vi "daqio_Re-Connect_Device.vi"(6 "re-connect timeouts":u32=1000, 7 "Credentials":T4, 8 "error in":errorcluster, 9 "override any errors":bool, 10 "re-connect attempts":i32=5, 11 "daq.io type in":T2={"daq.io ref"=refnum, "daq.io API Base"="http://dashboard.daq.io/api/v1", "Device Type Key"="", "Device Key"="", "Account ID"="", "online"=FALSE}) -> (0 "error out":errorcluster, 2 "status":T1, 3 "daq.io type out":T2={"daq.io ref"=refnum, "daq.io API Base"="http://dashboard.daq.io/api/v1", "Device Type Key"="", "Device Key"="", "Account ID"="", "online"=FALSE})   [LabVIEW 2013, in "daqio minimal.lvlib"]
doc: "This VI tries to re-connect the current device (the one the VI is executed on) to the daq.io cloud connection.\n\nThis VI can use multiple attempts to re-connect to the cloud. On Vxworks targets such as CompactRIO and SingleBoard RIO systems, this check may result in a timed out http GET function that can block the execution of code, therefore please run it in parallel and share the connection data globally by queue or FGV."
uses:
  daqio minimal.lvlib
  _typedefs/daqio-Credentials.ctl
  _typedefs/daqio-Type.ctl
  <vilib>/httpClient/ClientHandle.ctl
  _typedefs/daqio-reconnect-status.ctl
  <vilib>/httpClient/LabVIEWHTTPClient.lvlib
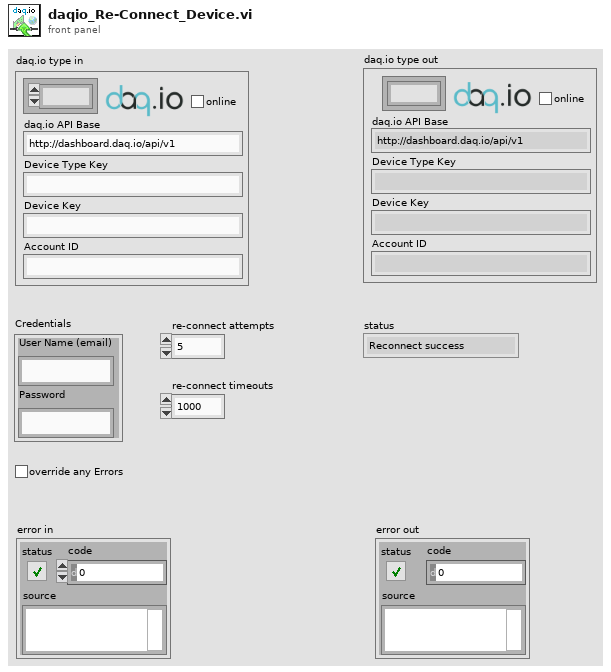
[diagram p1: front panel]
types:
  T1 = typedef "daqio minimal.lvlib/daqio-reconnect-status.ctl" = enum16{"Reconnect success", "Reconnect failed", "Connected"}
  T2 = typedef "daqio minimal.lvlib/daqio-Type.ctl" = cluster{"daq.io ref":T3, "daq.io API Base":string, "Device Type Key":string, "Device Key":string, "Account ID":string, "online":bool}
  T3 = typedef "LabVIEWHTTPClient.lvlib/ClientHandle.ctl" = refnum<k1>
  T4 = typedef "daqio minimal.lvlib/daqio-Credentials.ctl" = cluster{"User Name (email)":string, "Password":string}
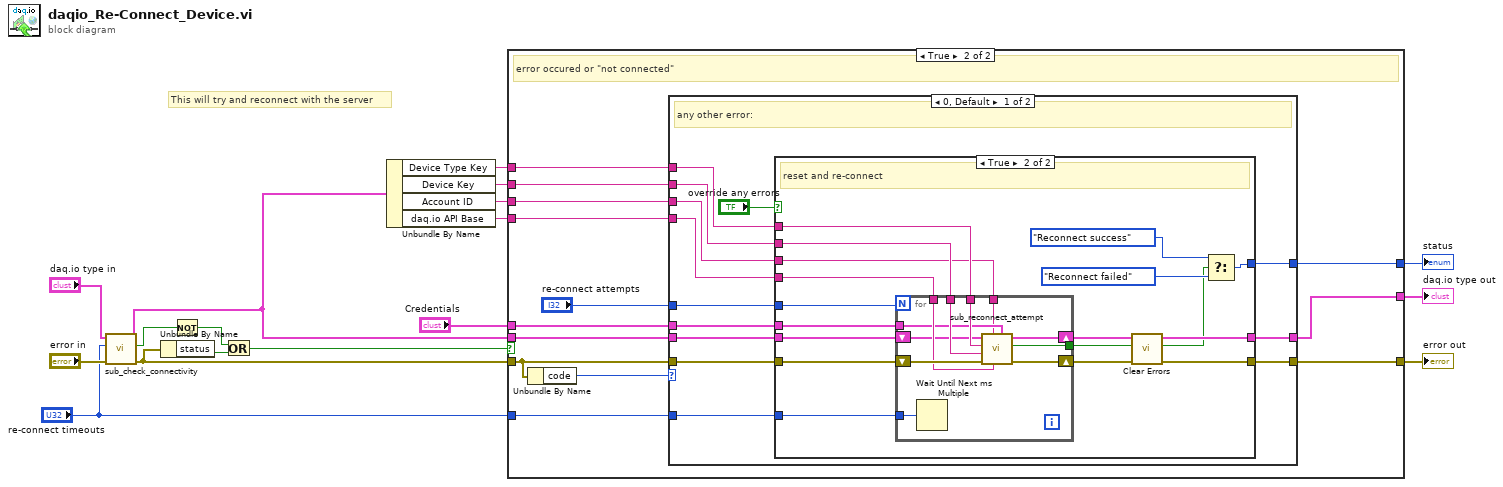
[diagram p0: block diagram]
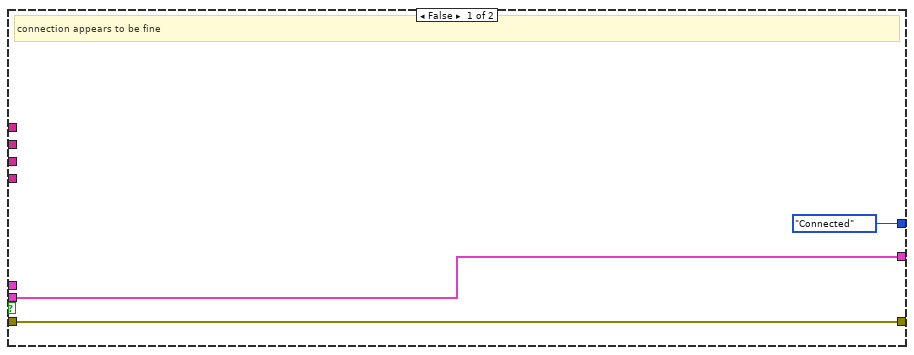
[diagram p2: hidden frame]
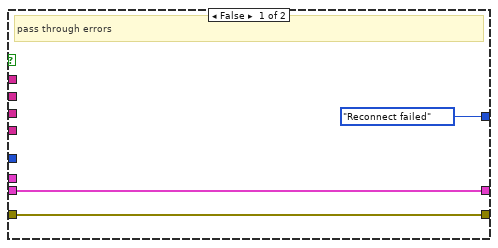
[diagram p3: hidden frame]
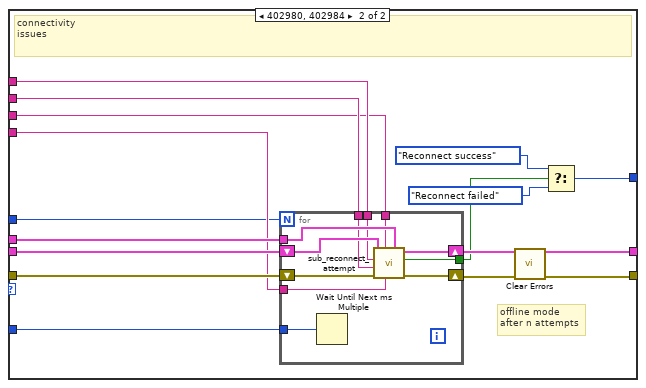
[diagram p4: hidden frame]
diagram:
  # "This will try and reconnect with the server"
  n1 = call "sub_check_connectivity.vi"("error in (no error)"="error in", "timeout (1000)"="re-connect timeouts", "daq.io type in"="daq.io type in") -> ("error out"=w3:errorcluster, "connected"=w2:bool, "daq.io type out"=w5:T2)  [unwired: 6 in]
  n2 = Unbundle By Name(w3) -> ("status"=w14:bool)
  n3 = Not(x=w2) -> (.not. x?=w15:bool)
  n4 = Or(x=w15, y=w14) -> (x .or. y?=w13:bool)
  n5 = Unbundle By Name(w5) -> ("Device Type Key"=w11:string, "Device Key"=w10:string, "Account ID"=w6:string, "daq.io API Base"=w7:string)
  n6 = case shown="True" w13 {
    tunnel: w3 -> [w19 w32]
    tunnel: "Credentials" -> [_ w31]
    tunnel: w11 -> [_ w30]
    tunnel: w10 -> [_ w29]
    tunnel: [w20 w28] -> w9
    tunnel: [w19 w27] -> w8
    tunnel: w5 -> [w20 w26]
    tunnel: w7 -> [_ w25]
    tunnel: w6 -> [_ w24]
    tunnel: [daqio-reconnect-status."Connected" ("status 2") w22] -> w4
    tunnel: "re-connect timeouts" -> [_ w21]
    frame False {
      # "connection appears to be fine"
    }
    frame True {
      # "error occured or \"not connected\""
      n7 = Unbundle By Name(w32) -> ("code"=w33:i32)
      n8 = case shown="0, Default" w33 {
        tunnel: w32 -> [w45 w88]
        tunnel: w31 -> [w44 w91]
        tunnel: w30 -> [w42 w90]
        tunnel: w29 -> [w43 w89]
        tunnel: [w41 w85] -> w28
        tunnel: [w40 w81] -> w27
        tunnel: w26 -> [w39 w92]
        tunnel: w25 -> [w38 w86]
        tunnel: w24 -> [w37 w87]
        tunnel: "re-connect attempts" -> [w36 w84]
        tunnel: w21 -> [w35 w83]
        tunnel: [w34 w82] -> w22
        frame 0, Default {
          # "any other error:"
          n9 = case shown="True" "override any errors" {
            tunnel: w45 -> [w49 w65]
            tunnel: w44 -> [_ w60]
            tunnel: w43 -> [_ w63]
            tunnel: w42 -> [_ w62]
            tunnel: [w48 w58] -> w41
            tunnel: [w49 w54] -> w40
            tunnel: w39 -> [w48 w61]
            tunnel: w38 -> [_ w64]
            tunnel: w37 -> [_ w59]
            tunnel: w36 -> [_ w57]
            tunnel: w35 -> [_ w56]
            tunnel: [daqio-reconnect-status."Reconnect failed" ("status 2") w55] -> w34
            frame False {
              # "pass through errors"
            }
            frame True {
              # "reset and re-connect"
              n10 = for {
                N: w57 -> [_]
                tunnel: w64 -> [w74]
                tunnel: w63 -> [w73]
                tunnel: w62 -> [w72]
                tunnel: w60 -> [w70]
                tunnel: w59 -> [w69]
                tunnel: [w68] -> w50
                shift-right: [w76] -> w51
                shift-left: w65 -> [w75]
                shift-right: [w67] -> w58
                shift-left: w61 -> [w71]
                tunnel: w56 -> [w66]
                n11 = Wait Until Next ms Multiple(millisecond multiple=w66) -> ()  [unwired: 1 out]
                n12 = call "sub_reconnect_attempt.vi"("Credentials"=w70, "daq.io API Base"=w74, "Account ID"=w69, "error in (no error)"=w75, "Device Key"=w73, "Device Type Key"=w72, "daq.io type in OLD"=w71) -> ("error out"=w76:errorcluster, "logged in?"=w68:bool, "daq.io type out"=w67:T2)  [unwired: 2 in]
              }
              n13 = call <vilib>:"Clear Errors.vi"("error in (no error)"=w51) -> ("error out"=w54:errorcluster)  [unwired: 6 in]
              n14 = Select(t=daqio-reconnect-status."Reconnect success" ("status 2"), s=w50, f=daqio-reconnect-status."Reconnect failed" ("status 2")) -> (s? t:f=w55:T1)
            }
          }
        }
        frame 402980, 402984 {
          # "offline mode\nafter n attempts"
          # "connectivity\nissues"
          n15 = for {
            N: w84 -> [_]
            tunnel: w91 -> [w102]
            tunnel: w90 -> [w101]
            tunnel: w89 -> [w100]
            tunnel: w87 -> [w98]
            tunnel: w86 -> [w97]
            tunnel: [w94] -> w77
            shift-right: [w93] -> w78
            shift-left: w88 -> [w99]
            shift-right: [w96] -> w85
            shift-left: w92 -> [w103]
            tunnel: w83 -> [w95]
            n16 = Wait Until Next ms Multiple(millisecond multiple=w95) -> ()  [unwired: 1 out]
            n17 = call "sub_reconnect_attempt.vi"("Credentials"=w102, "daq.io API Base"=w97, "Account ID"=w98, "error in (no error)"=w99, "Device Key"=w100, "Device Type Key"=w101, "daq.io type in OLD"=w103) -> ("error out"=w93:errorcluster, "logged in?"=w94:bool, "daq.io type out"=w96:T2)  [unwired: 2 in]
          }
          n18 = call <vilib>:"Clear Errors.vi"("error in (no error)"=w78) -> ("error out"=w81:errorcluster)  [unwired: 6 in]
          n19 = Select(t=daqio-reconnect-status."Reconnect success" ("status 2"), s=w77, f=daqio-reconnect-status."Reconnect failed" ("status 2")) -> (s? t:f=w82:T1)
        }
      }
    }
  }
  "error out" <- w8
  "daq.io type out" <- w9
  "status" <- w4
